vi "Report Event.vi"(7 "Level (Info)":T1=enum."Info", 8 "error in (no error)":errorcluster, 9 "Message":string, 10 "Context":string, 11 "VolatusAPI in":refnum<class "VolatusAPI.lvclass">) -> (0 "error out":errorcluster, 3 "VolatusAPI out":refnum<class "VolatusAPI.lvclass">)   [LabVIEW 2020, in "Volatus.lvlib" / "VolatusAPI.lvclass"]
uses:
  VolatusAPI.lvclass
  Event Level.ctl
  VolatusAPI.lvclass/VolatusAPI.ctl
  Volatus.lvlib
  Event.ctl
  MessageQ/MessageQ.lvclass
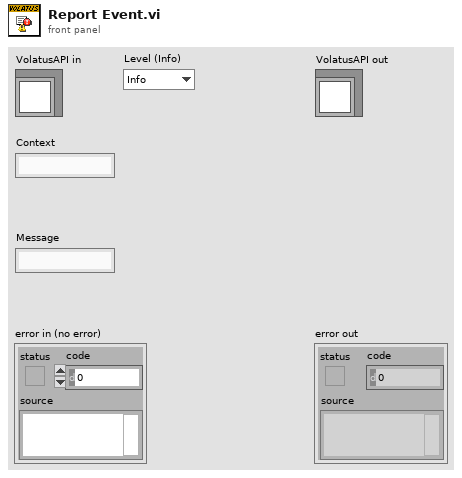
[diagram p1: front panel]
types:
  T1 = typedef "Volatus.lvlib/Event Level.ctl" = enum16{"Debug", "Info", "Warning", "Error"}
  T2 = typedef "Volatus.lvlib/Event.ctl" = cluster{"Time Stamp":timestamp, "Event Level":T1, "Context":string, "Message":string, "Error":errorcluster}
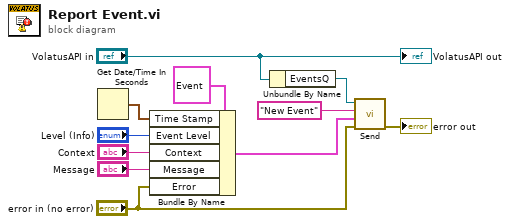
[diagram p0: block diagram]
diagram:
  n1 = Get Date/Time In Seconds() -> (seconds since 1Jan1904=w1:timestamp)
  n2 = Bundle By Name(cluster=T2 {"Time Stamp"=timestamp(0 s since 1904-01-01), "Event Level"=enum."Info", "Context"="", "Message"="", "Error"={"status"=FALSE, "code"=0, "source"=""}} ("Event"), "Time Stamp"=w1, "Event Level"="Level (Info)", "Context"="Context", "Message"="Message", "Error"="error in (no error)") -> (w4:T2)
  n3 = Unbundle By Name("VolatusAPI in") -> ("EventsQ"=w6:refnum<class "MessageQ.lvclass">)
  n4 = call "Send.vi"("error in (no error)"="error in (no error)", "Data"=w4, "ID"="New Event", "MessageQ in"=w6) -> ("error out"=→"error out":errorcluster)  [unwired: 6 in, 1 out]
  "VolatusAPI out" <- "VolatusAPI in"
